vi "ReportError Event Callback.vi"(4 "User Parameter":variant, 5 "Event data":cluster{"errorCode":i32, "errorMessage":string}, 6 "CtlRef":refnum<k7>, 7 "Event common data":cluster{"Source":i32, "Type":u32, "Time":u32}) -> ()   [LabVIEW 2010, in "TS Simple LabVIEW OI Dependencies.lvlib"]
uses:
  TS Simple LabVIEW OI Dependencies.lvlib
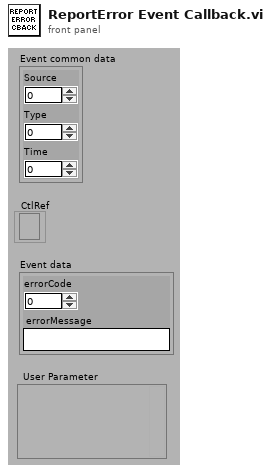
[diagram p1: front panel]
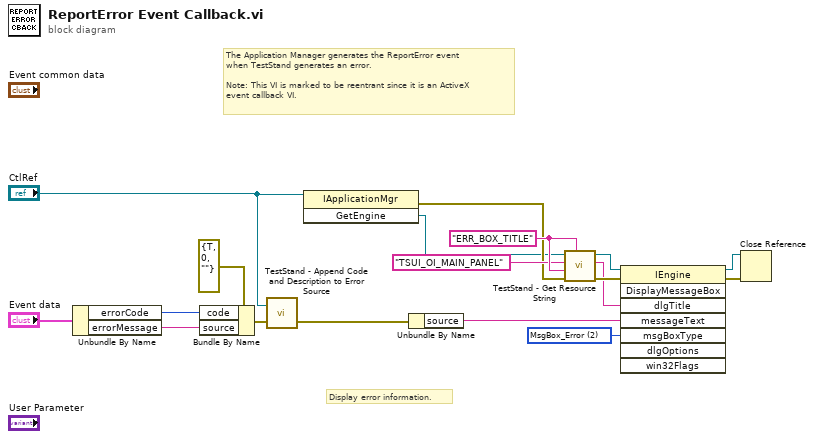
[diagram p0: block diagram]
diagram:
  w7 = 2 items=["MsgBox_Warning", "MsgBox_Information", "MsgBox_Error", "MsgBox_Custom"] ("msgBoxType")
  w10 = "ERR_BOX_TITLE" ("Symbol")
  # "Display error information."
  # "The Application Manager generates the ReportError event\nwhen TestStand generates an error.\n\nNote: This VI is marked to be reentrant since it is an ActiveX\nevent callback VI."
  n1 = Unbundle By Name("Event data") -> ("errorCode"=w16:i32, "errorMessage"=w17:string)
  n2 = Bundle By Name(cluster=errorcluster {"status"=TRUE, "code"=0, "source"=""} ("error in (no error)"), "code"=w16, "source"=w17) -> (w14:errorcluster)
  n3 = call <vilib>:"TestStand - Append Code and Description to Error Source.vi"("error in (no error)"=w14, "Application Manager Ref In"="CtlRef") -> ("error out"=w6:errorcluster)  [unwired: 1 out]
  n4 = invoke class="IApplicationMgr" method="GetEngine"(reference="CtlRef") -> (error out=w4:errorcluster, "GetEngine"=w3:refnum<k7>)  [unwired: 2 in, 1 out]
  n5 = Unbundle By Name(w6) -> ("source"=w8:string)
  n6 = call <vilib>:"TestStand - Get Resource String.vi"("Default String"=w10, "error in (no error)"=w4, "Symbol"=w10, "Category"="TSUI_OI_MAIN_PANEL", "Engine Reference In"=w3) -> ("error out"=w13:errorcluster, "Resource String"=w11:string, "Engine Reference Out"=w12:refnum<k7>)  [unwired: 4 out]
  n7 = invoke class="IEngine" method="DisplayMessageBox"(reference=w12, error in=w13, "dlgTitle"=w11, "messageText"=w8, "msgBoxType"=w7) -> (reference out=w1:refnum<k7>, error out=w2:errorcluster)  [unwired: 3 in, 6 out]
  n8 = Close Reference(reference=w1, error in (no error)=w2) -> ()  [unwired: 1 out]
